vi "Configure OPP.vi"(8 "error in (no error)":errorcluster, 10 "Power Limit (150.00 W)":dbl=150.0 min=0.0 max=1500.0 step=0.01 format="%.2g", 11 "VISA resource name":refnum<visa-resource-name>) -> (0 "error out":errorcluster, 3 "VISA resource name out":refnum<visa-resource-name>)   [LabVIEW 2019, in "BK Precision 8500B Series.lvlib"]
doc: "Configures over power protection (OPP)."
uses:
  <instrlib>/BK Precision 8500B Series/BK Precision 8500B Series.lvlib
panel:
  # "W"
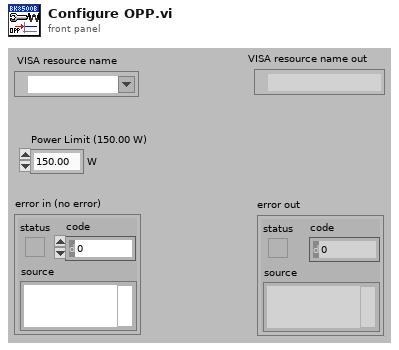
[diagram p1: front panel]
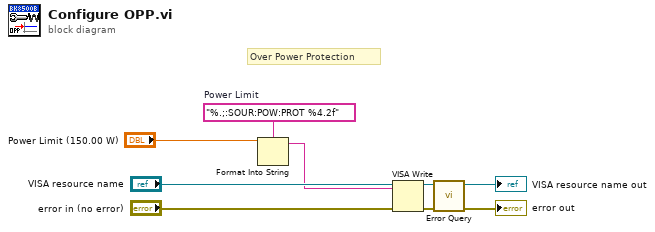
[diagram p0: block diagram]
diagram:
  w9 = "%.;:SOUR:POW:PROT %4.2f"  # Power Limit
  # "Over Power Protection"
  n1 = Format Into String(format string=w9, "Power Limit (150.00 W)") -> (resulting string=w1:string)  [unwired: 2 in, 1 out]
  n2 = VISA Write(VISA resource name="VISA resource name", write buffer=w1, error in (no error)="error in (no error)") -> (VISA resource name out=w7:refnum<visa-resource-name>, error out=w6:errorcluster)  [unwired: 1 out]
  n3 = call <instrlib>:"Error Query.vi"("error in (no error)"=w6, "VISA resource name"=w7) -> ("error out"=→"error out":errorcluster, "VISA resource name out"=→"VISA resource name out":refnum<visa-resource-name>)  [unwired: 6 in, 2 out]
